vi "SerializeInsertMeasurement.vi"(3 "error in (no error)":errorcluster, 4 "InsertMeasurement":T1, 5 "LotData in":refnum<class "LotData.lvclass">) -> (0 "error out":errorcluster, 1 "Json":string, 2 "LotData out":refnum<class "LotData.lvclass">)   [LabVIEW 2012, in "LotData.lvclass"]
uses:
  LotData.lvclass
  Controls/JsonTypes/InsertMeasurement.ctl
  Controls/MeasurementType.ctl
  <vilib>/LVH/i3 JSON/JSON Generation/Create Value Files/Create Value - Object.vi
  <vilib>/LVH/i3 JSON/JSON Generation/Add Object Parameter Files/Add Object Parameter - String.vi
  <vilib>/LVH/i3 JSON/JSON Generation/Add Object Parameter Files/Add Object Parameter - Numeric.vi
  <vilib>/LVH/i3 JSON/i3-json.lvlib
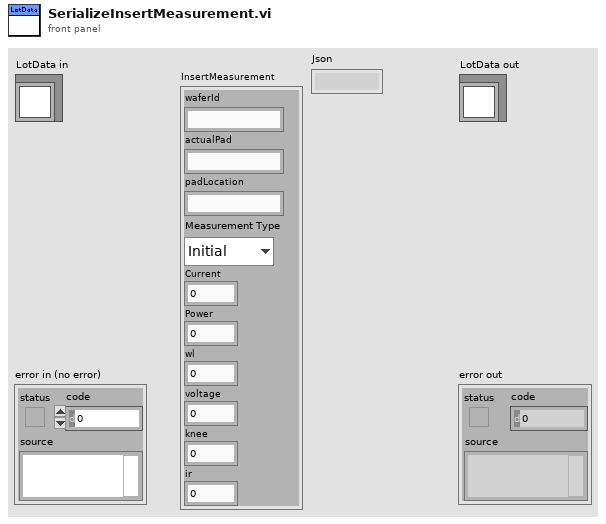
[diagram p1: front panel]
types:
  T1 = typedef "InsertMeasurement.ctl" = cluster{"waferId":string, "actualPad":string, "padLocation":string, "Measurement Type":T2, "Current":dbl, "Power":dbl, "wl":dbl, "voltage":dbl, "knee":dbl, "ir":dbl}
  T2 = typedef "MeasurementType.ctl" = enum16{"Initial", "Final"}
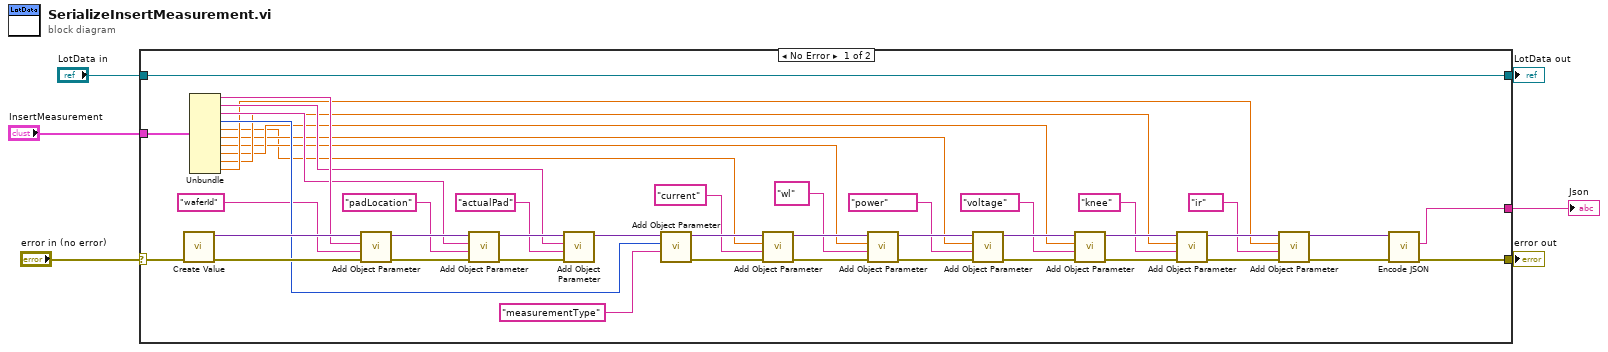
[diagram p0: block diagram]
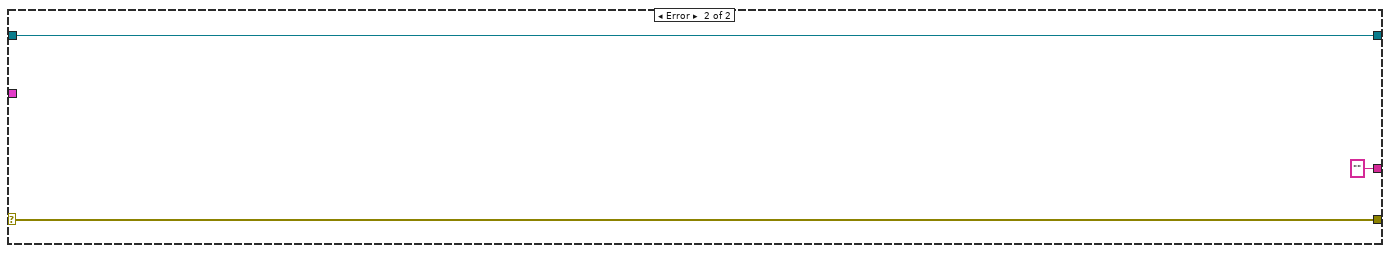
[diagram p2: hidden frame]
diagram:
  n1 = case shown="No Error" "error in (no error)" {
    selector: "error in (no error)" -> [w51 w55]
    tunnel: [w8 w55] -> w5
    tunnel: [w52 w54] -> w3
    tunnel: "LotData in" -> [w52 w54]
    tunnel: "InsertMeasurement" -> [w46 _]
    tunnel: [w7 "" ("String")] -> w1
    frame No Error {
      n2 = call-poly <vilib>:"Create Value.vi"("error in (no error)"=w51) -> ("error out"=w49:errorcluster, "JSON Tree"=w50:variant)  [unwired: 9 in]
      n3 = Unbundle(w46) -> ("waferId"=w45:string, "actualPad"=w35:string, "padLocation"=w36:string, "Measurement Type"=w43:T2, "Current"=w11:dbl, "Power"=w13:dbl, "wl"=w12:dbl, "voltage"=w14:dbl, "knee"=w15:dbl, "ir"=w16:dbl)
      n4 = call-poly <vilib>:"Add Object Parameter.vi"("error in (no error)"=w49, "Name"="waferId", "String"=w45, "JSON Tree in (JSON Object)"=w50) -> ("error out"=w39:errorcluster, "JSON Tree out (JSON Object)"=w48:variant)  [unwired: 6 in]
      n5 = call-poly <vilib>:"Add Object Parameter.vi"("error in (no error)"=w39, "Name"="padLocation", "String"=w36, "JSON Tree in (JSON Object)"=w48) -> ("error out"=w40:errorcluster, "JSON Tree out (JSON Object)"=w47:variant)  [unwired: 6 in]
      n6 = call-poly <vilib>:"Add Object Parameter.vi"("error in (no error)"=w40, "Name"="actualPad", "String"=w35, "JSON Tree in (JSON Object)"=w47) -> ("JSON Tree out (JSON Object)"=w44:variant)  [unwired: 6 in, 1 out]
      n7 = call-poly <vilib>:"Add Object Parameter.vi"("Name"="measurementType", "Numeric"=w43, "JSON Tree in (JSON Object)"=w44) -> ("error out"=w17:errorcluster, "JSON Tree out (JSON Object)"=w29:variant)  [unwired: 7 in]
      n8 = call-poly <vilib>:"Add Object Parameter.vi"("error in (no error)"=w17, "Name"="current", "Numeric"=w11, "JSON Tree in (JSON Object)"=w29) -> ("error out"=w18:errorcluster, "JSON Tree out (JSON Object)"=w30:variant)  [unwired: 6 in]
      n9 = call-poly <vilib>:"Add Object Parameter.vi"("error in (no error)"=w18, "Name"="wl", "Numeric"=w12, "JSON Tree in (JSON Object)"=w30) -> ("error out"=w19:errorcluster, "JSON Tree out (JSON Object)"=w31:variant)  [unwired: 6 in]
      n10 = call-poly <vilib>:"Add Object Parameter.vi"("error in (no error)"=w19, "Name"="power", "Numeric"=w13, "JSON Tree in (JSON Object)"=w31) -> ("error out"=w20:errorcluster, "JSON Tree out (JSON Object)"=w32:variant)  [unwired: 6 in]
      n11 = call-poly <vilib>:"Add Object Parameter.vi"("error in (no error)"=w20, "Name"="voltage", "Numeric"=w14, "JSON Tree in (JSON Object)"=w32) -> ("error out"=w21:errorcluster, "JSON Tree out (JSON Object)"=w33:variant)  [unwired: 6 in]
      n12 = call-poly <vilib>:"Add Object Parameter.vi"("error in (no error)"=w21, "Name"="knee", "Numeric"=w15, "JSON Tree in (JSON Object)"=w33) -> ("error out"=w22:errorcluster, "JSON Tree out (JSON Object)"=w34:variant)  [unwired: 6 in]
      n13 = call-poly <vilib>:"Add Object Parameter.vi"("error in (no error)"=w22, "Name"="ir", "Numeric"=w16, "JSON Tree in (JSON Object)"=w34) -> ("error out"=w9:errorcluster, "JSON Tree out (JSON Object)"=w10:variant)  [unwired: 6 in]
      n14 = call <vilib>:"Encode JSON.vi"("error in (no error)"=w9, "JSON Tree"=w10) -> ("error out"=w8:errorcluster, "String"=w7:string)  [unwired: 4 in]
    }
    frame Error {
    }
  }
  "error out" <- w5
  "LotData out" <- w3
  "Json" <- w1
